vi "Remove VI.vi"(8 "error in":errorcluster, 10 "VI names":string[](array[string]), 11 "state in":T1) -> (0 "error out":errorcluster, 1 "removed?":bool, 3 "state out":T1)   [LabVIEW 2010, in "NI_SE_Config Front Panel Layout.lvlib"]
uses:
  NI_SE_Config Front Panel Layout.lvlib
  State.ctl
  VI Info.ctl
  VI Panel Layout/VI Panel Layout.lvclass
  VI Panel Layout/VI Panel Layout.lvclass/VI Panel Layout.ctl
  VI Panel Layout/Get VI Name.vi
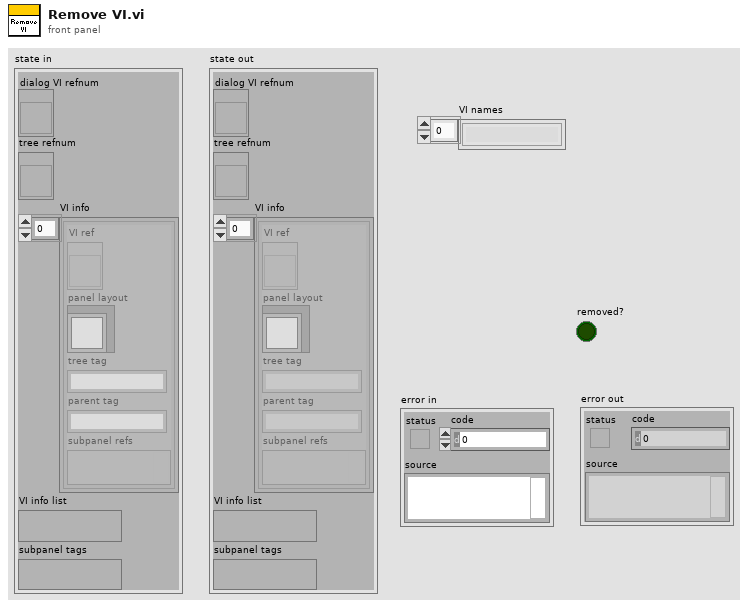
[diagram p1: front panel]
types:
  T1 = typedef "NI_SE_Config Front Panel Layout.lvlib/State.ctl" = cluster{"dialog VI refnum":refnum<vi>, "tree refnum":refnum<vi>, "VI info":T2[], "VI info list":variant, "subpanel tags":variant}
  T2 = typedef "NI_SE_Config Front Panel Layout.lvlib/VI Info.ctl" = cluster{"VI ref":refnum<vi>, "panel layout":refnum<class "VI Panel Layout.lvclass">, "tree tag":string, "parent tag":string, "subpanel refs":variant}
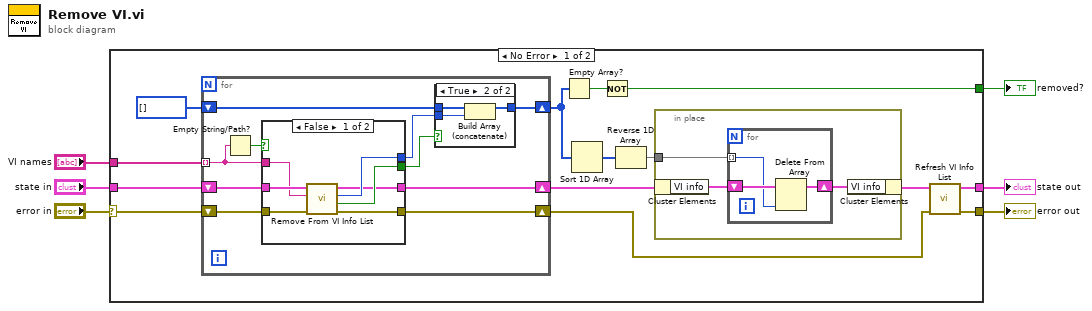
[diagram p0: block diagram]
diagram:
  n1 = case shown="No Error" "error in" {
    selector: "error in" -> [w18 w50]
    tunnel: "state in" -> [w19 w51]
    tunnel: [w13 w51] -> w4
    tunnel: [w11 w50] -> w3
    tunnel: "VI names" -> [w20 _]
    tunnel: [w8 _] -> w1
    frame No Error {
      n2 = for {
        tunnel: w20 -> [w35] mode=indexing
        shift-right: [w32] -> w15
        shift-left: w19 -> [w34]
        shift-right: [w31] -> w12
        shift-left: w18 -> [w33]
        shift-right: [w27] -> w10
        shift-left: i32[] [] ("Array") -> [w28]
        n3 = Empty String/Path?(string/path=w35) -> (empty?=w36:bool)
        n4 = case shown="False" w36 {
          tunnel: w35 -> [w45 _]
          tunnel: w34 -> [w47 w49]
          tunnel: w33 -> [w46 w48]
          tunnel: [w41 w49] -> w32
          tunnel: [w42 w48] -> w31
          tunnel: [w44 _] -> w30
          tunnel: [w43 _] -> w29
          frame False {
            n5 = call "Remove From VI Info List.vi"("error in"=w46, "VI name"=w45, "state in"=w47) -> ("error out"=w42:errorcluster, "found?"=w43:bool, "VI info index"=w44:i32, "state out"=w41:T1)  [unwired: 5 in]
          }
          frame True {
          }
        }
        n6 = case shown="True" w29 {
          tunnel: w28 -> [w37 w39]
          tunnel: w30 -> [_ w38]
          tunnel: [w37 w40] -> w27
          frame False {
          }
          frame True {
            n7 = Build Array (concatenate)(w39, w38) -> (w40:i32[])
          }
        }
      }
      n8 = Empty Array?(array=w10) -> (empty?=w9:bool)
      n9 = Sort 1D Array(array=w10) -> (sorted array=w17:i32[])
      n10 = Not(x=w9) -> (.not. x?=w8:bool)
      n11 = Reverse 1D Array(array=w17) -> (reversed array=w16:i32[])
      n12 = in-place {
        in-place-border: w16 -> [w23]
        n13 = in-place-cluster #1(w15) -> ("VI info"=w22:T2[])
        n14 = for {
          tunnel: w23 -> [w25] mode=indexing
          shift-right: [w24] -> w21
          shift-left: w22 -> [w26]
          n15 = Delete From Array(array=w26, index=w25) -> (array with subset deleted=w24:T2[])  [unwired: 1 in, 1 out]
        }
        n16 = in-place-cluster #1("VI info"=w21) -> (w14:T1)
      }
      n17 = call "Refresh VI Info List.vi"("error in"=w12, "state in"=w14) -> ("error out"=w11:errorcluster, "state out"=w13:T1)  [unwired: 8 in]
    }
    frame Error {
    }
  }
  "state out" <- w4
  "error out" <- w3
  "removed?" <- w1
